vi "ReadPXI-6229Tasks.vi"(8 "Error In":errorcluster, 11 "PXI-6229 Tasks In":refnum<k21>[](array[refnum])) -> (0 "Error Out":errorcluster, 2 "PXI-6229 Data":T1, 3 "PXI-6229 Tasks Out":refnum<k21>[](array[refnum]))   [LabVIEW 2012]
uses:
  PXI6229Data.ctl
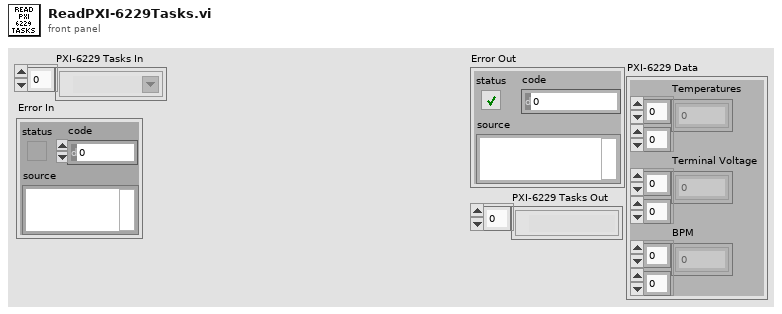
[diagram p1: front panel]
types:
  T1 = typedef "PXI6229Data.ctl" = cluster{"Temperatures":dbl[][], "Terminal Voltage":dbl[][], "BPM":dbl[][]}
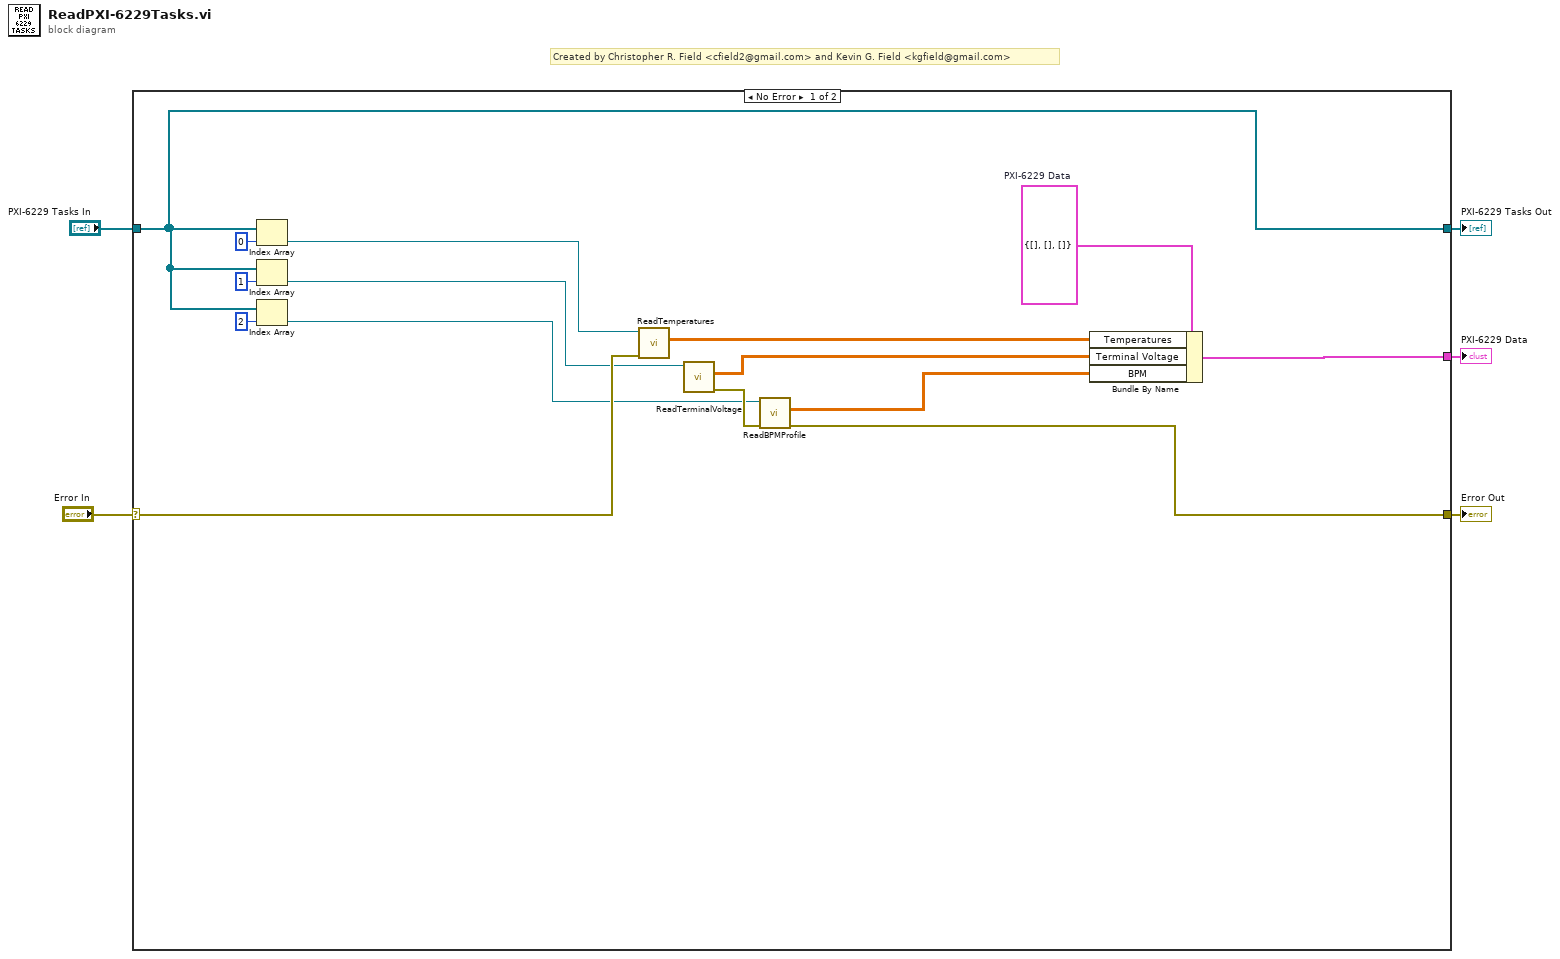
[diagram p0: block diagram]
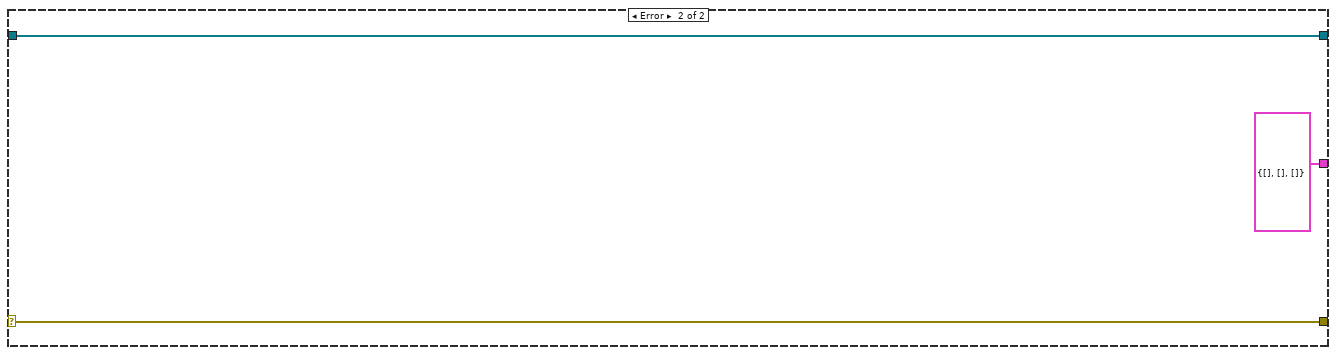
[diagram p2: hidden frame]
diagram:
  # "Created by Christopher R. Field <cfield2@gmail.com> and Kevin G. Field <kgfield@gmail.com>"
  n1 = case shown="No Error" "Error In" {
    selector: "Error In" -> [w19 w23]
    tunnel: "PXI-6229 Tasks In" -> [w10 w21]
    tunnel: [w18 w23] -> w3
    tunnel: [w11 T1 {"Temperatures"=[], "Terminal Voltage"=[], "BPM"=[]} ("DAQ Data Queue Element")] -> w2
    tunnel: [w10 w21] -> w1
    frame No Error {
      w13 = T1 {"Temperatures"=[], "Terminal Voltage"=[], "BPM"=[]}  # PXI-6229 Data
      n2 = Index Array(array=w10, index=0) -> (element=w14:refnum<k21>)
      n3 = Index Array(array=w10, index=1) -> (element=w9:refnum<k21>)
      n4 = Index Array(array=w10, index=2) -> (element=w8:refnum<k21>)
      n5 = call "ReadTemperatures.vi"("Error In"=w19, "Temperature Task In"=w14) -> ("Raw Data"=w12:dbl[][])  [unwired: 7 in, 2 out]
      n6 = call "ReadTerminalVoltage.vi"("Terminal Voltage Task In"=w9) -> ("Error Out"=w20:errorcluster, "Raw Data"=w7:dbl[][])  [unwired: 8 in, 1 out]
      n7 = call "ReadBPMProfile.vi"("Error In"=w20, "BPM Task In"=w8) -> ("Error Out"=w18:errorcluster, "BPM Profile Data"=w6:dbl[][])  [unwired: 7 in, 1 out]
      n8 = Bundle By Name(cluster=w13, "Temperatures"=w12, "Terminal Voltage"=w7, "BPM"=w6) -> (w11:T1)
    }
    frame Error {
    }
  }
  "Error Out" <- w3
  "PXI-6229 Data" <- w2
  "PXI-6229 Tasks Out" <- w1
